vi "DefensorManMark.vi"(8 "AI Parameters":T1={"GotoKick"={"Dist do cone a frente"=150.0, "attacker farback"=1500.0, "Perto"=300.0, "min dist to kick"=150.0, "kick eps"=0.0, "Time to transition"=0.05}, "Attacker"={"CC chute"=0.09, "CC passe"=0.045, "Kick Force"=100.0, "D ball-robot Kick"=200.0, "D ball-robot Pass"=0.3}, "Defender"={"D max"=1700.0, "Vel p/ robô av"=1000.0, "Kick Force"=100.0, "D atk-def"=0.0, "D farback"=0.0}, "Timeout"={"Field/v in x"=6.0, "Dist Robots"=300, "Dist up in y"=300}, "Pose Striker"={"dist"=200.0, "Numeric"=-4.0, "dist 2"=200.0}, "Dist Stop"=300.0, "Distance when ball out"=200, "D central gap "=150.0, "T pass"=0.0, "Force ++"=0.0, "range kick"=0.0, "Chute alto"=TRUE, "Marcador novo"=TRUE} {"D central gap" format="%#_13g"; "Dist Stop" format="%#_13g"; "Pose Striker"."Numeric" format="%#_13g"; "Defender"."Kick Force" format="%#_13g"; "Defender"."Vel p/ robô av" format="%#_13g"; "Attacker"."D ball-robot Kick" format="%#_13g"; "Attacker"."Kick Force" format="%#_13g"; "Attacker"."CC passe" format="%#_13g"; "Attacker"."CC chute" format="%#_13g"; "GotoKick"."kick eps" format="%#_13g"; "GotoKick"."min dist to kick" format="%#_13g"; "GotoKick"."Perto" format="%#_13g"; "GotoKick"."attacker farback" format="%#_13g"; "GotoKick"."Dist do cone a frente" format="%#_13g"}, 9 "Robot in":T3={"id"=5, "function"=enum."Attacker", "x"=-1842.5054931640625, "y"=520.60986328125, "orientation"=-2.7555055618286133, "v_tangent"=0.0, "v_normal"=0.0, "v_ang"=0.0, "kick_x"=0.0, "kick_z"=0.0, "dribble"=FALSE, "Timestamp"=timestamp(2082758857.4639893 s since 1904-01-01), "estimatives"={"est_v_tangent"=0.0, "est_v_normal"=0.0, "est_vx"=0.0, "est_vy"=0.0, "Pos Robot Est"=[]}, "dest_x_kick"=0.0, "dest_y_kick"=0.0, "Gap Coord"=[], "States"=enum."GoToTangent", "Path "=[], "Path  Smooth"=[], "Dest"=[]}, 10 "Field Size in":T9, 11 "IA Input":T2={"our_robots"=[], "enemy_robots"=[], "balls"=[], "geometry"={"line_width"=0, "field_length"=0, "field_width"=0, "boundary_width"=0, "referee_width"=0, "goal_width"=0, "goal_depth"=0, "goal_wall_width"=0, "center_circle_radius"=0, "defense_radius"=0, "defense_stretch"=0, "free_kick_from_defense_dist"=0, "penalty_spot_from_field_line_dist"=0, "penalty_line_from_spot_dist"=0}, "IA Judge"={"stage"="", "command"="", "our_goalie_id"=0.0, "enemy_goalie_id"=0.0, "command enum"=enum."Halt", "Time"=enum."Azul"}, "Received Timestamp"=timestamp(0 s since 1904-01-01), "Events"={"Touch"=FALSE, "Ball out"=FALSE, "id touch"=0.0, "Ball out of \nVision"=FALSE, "Ball inside \nGoalie area"=FALSE, "Robot not responding"=FALSE, "Robots responding status"=[1.0, 1.0, 1.0, 1.0, 1.0, 1.0], "Enemy Ball \nPossession"=FALSE, "Pass State"=FALSE, "id end of pass"=0.0, "Kick"=FALSE, "Id ini Possession"=0.0, "Ball Possesion"=FALSE, "Id Possesion"=0.0}}) -> (2 "Robot out":T3={"id"=0, "function"=enum."Attacker", "x"=0.0, "y"=0.0, "orientation"=0.0, "v_tangent"=0.0, "v_normal"=0.0, "v_ang"=0.0, "kick_x"=0.0, "kick_z"=0.0, "dribble"=FALSE, "Timestamp"=timestamp(0 s since 1904-01-01), "estimatives"={"est_v_tangent"=0.0, "est_v_normal"=0.0, "est_vx"=0.0, "est_vy"=0.0, "Pos Robot Est"=[]}, "dest_x_kick"=0.0, "dest_y_kick"=0.0, "Gap Coord"=[], "States"=enum."GoToTangent", "Path "=[], "Path  Smooth"=[], "Dest"=[]}, 3 "id do inimigo\nmais perigoso":u32)   [LabVIEW 2017]
uses:
  Core/Field Size.ctl
  Core/AI Robot.ctl
  Functions Enum.ctl
  AttackerStates.ctl
  Path Planning/RRT/PathDests.ctl
  Path Planning/RRT/PathDest.ctl
  Core/AI Input.ctl
  Core/AI Ball.ctl
  Core/AI Judge.ctl
  Command Enum.ctl
  Util/Events/Events.ctl
  AI Parameters.ctl
  <vilib>/Analysis/_algsub.llb/Real Vector Norm.vi
  <vilib>/Analysis/NI_AALPro.lvlib
panel:
  in  "farback striker":dbl=500.0 format="%#_13g"
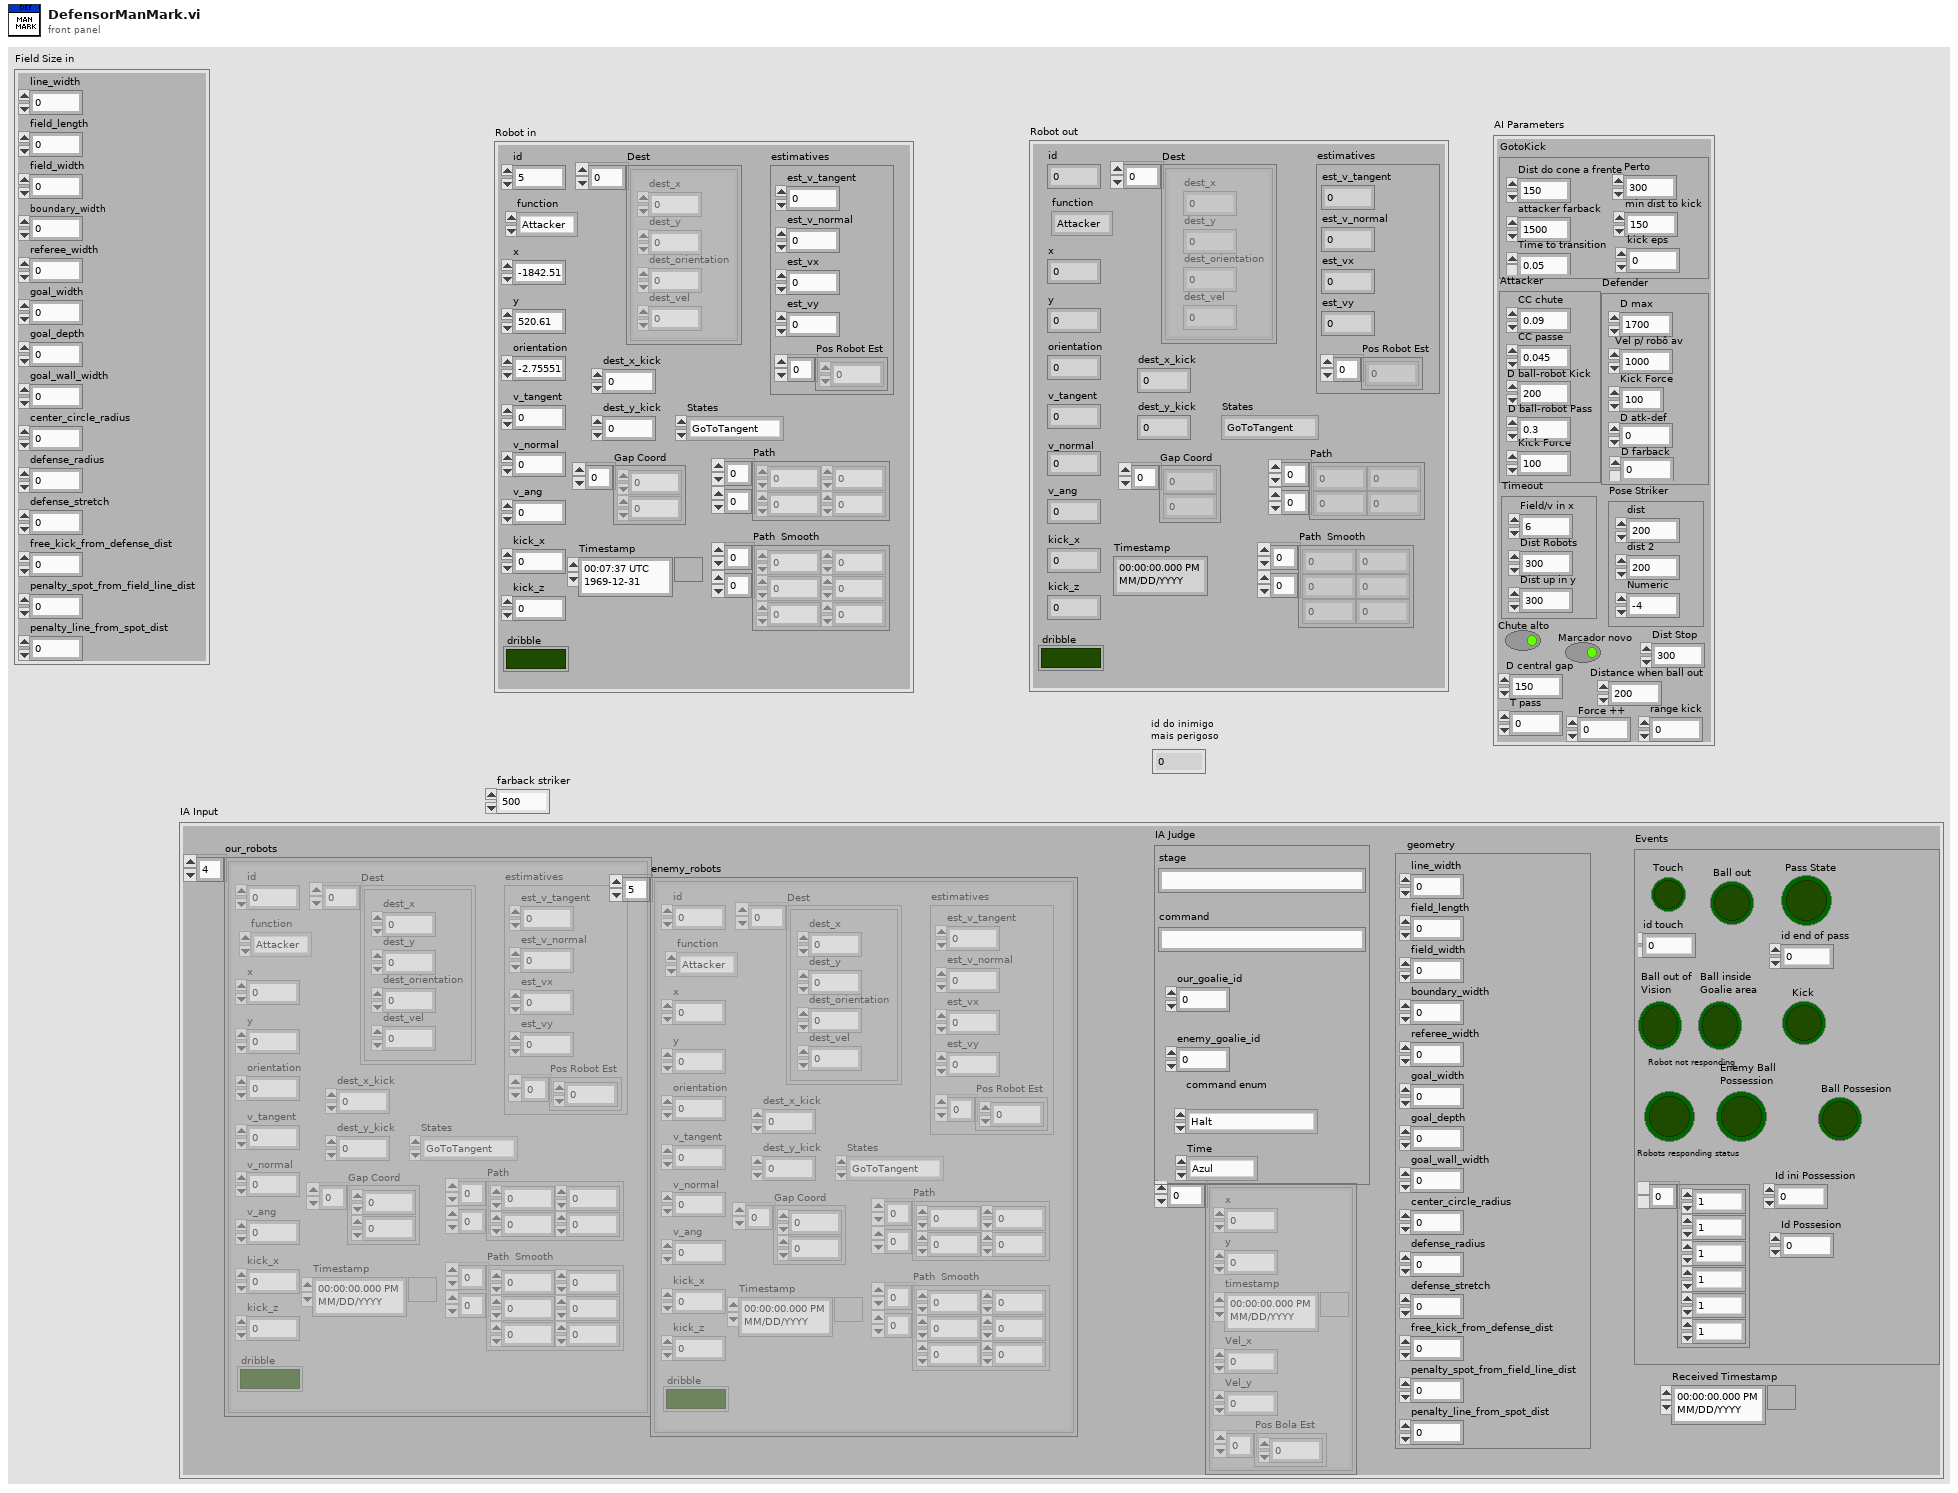
[diagram p1: front panel]
types:
  T1 = typedef "AI Parameters.ctl" = cluster{"GotoKick":cluster{"Dist do cone a frente":dbl, "attacker farback":dbl, "Perto":dbl, "min dist to kick":dbl, "kick eps":dbl, "Time to transition":dbl}, "Attacker":cluster{"CC chute":dbl, "CC passe":dbl, "Kick Force":dbl, "D ball-robot Kick":dbl, "D ball-robot Pass":dbl}, "Defender":cluster{"D max":dbl, "Vel p/ robô av":dbl, "Kick Force":dbl, "D atk-def":dbl, "D farback":dbl}, "Timeout":cluster{"Field/v in x":dbl, "Dist Robots":u32, "Dist up in y":u32}, "Pose Striker":cluster{"dist":dbl, "Numeric":dbl, "dist 2":dbl}, "Dist Stop":dbl, "Distance when ball out":i32, "D central gap ":dbl, "T pass":dbl, "Force ++":dbl, "range kick":dbl, "Chute alto":bool, "Marcador novo":bool}
  T2 = typedef "AI Input.ctl" = cluster{"our_robots":T3[], "enemy_robots":T3[], "balls":T8[], "geometry":T9, "IA Judge":T10, "Received Timestamp":timestamp, "Events":T12}
  T3 = typedef "AI Robot.ctl" = cluster{"id":u32, "function":T4, "x":dbl, "y":dbl, "orientation":dbl, "v_tangent":dbl, "v_normal":dbl, "v_ang":dbl, "kick_x":dbl, "kick_z":dbl, "dribble":bool, "Timestamp":timestamp, "estimatives":cluster{"est_v_tangent":dbl, "est_v_normal":dbl, "est_vx":dbl, "est_vy":dbl, "Pos Robot Est":dbl[]}, "dest_x_kick":dbl, "dest_y_kick":dbl, "Gap Coord":dbl[], "States":T5, "Path ":dbl[][], "Path  Smooth":dbl[][], "Dest":T6}
  T4 = typedef "Functions Enum.ctl" = enum16{"Attacker", "Goalie", "Defender", "Striker", "Goto 0", "Dummy", "Kicker", "ZigZag"}
  T5 = typedef "AttackerStates.ctl" = enum16{"Pass", "GoToTangent", "BallGetting", "GoToKick", ""}
  T6 = typedef "PathDests.ctl" = T7[]
  T7 = typedef "PathDest.ctl" = cluster{"dest_x":dbl, "dest_y":dbl, "dest_orientation":dbl, "dest_vel":dbl}
  T8 = typedef "AI Ball.ctl" = cluster{"x":dbl, "y":dbl, "timestamp":timestamp, "Vel_x":dbl, "Vel_y":dbl, "Pos Bola Est":dbl[]}
  T9 = typedef "Field Size.ctl" = cluster{"line_width":u32, "field_length":u32, "field_width":u32, "boundary_width":u32, "referee_width":u32, "goal_width":u32, "goal_depth":u32, "goal_wall_width":u32, "center_circle_radius":u32, "defense_radius":u32, "defense_stretch":u32, "free_kick_from_defense_dist":u32, "penalty_spot_from_field_line_dist":u32, "penalty_line_from_spot_dist":u32}
  T10 = typedef "AI Judge.ctl" = cluster{"stage":string, "command":string, "our_goalie_id":dbl, "enemy_goalie_id":dbl, "command enum":T11, "Time":enum16{"Azul", "Amarelo"}}
  T11 = typedef "Command Enum.ctl" = enum16{"Halt", "Stop", "Force Start", "PKA Normal Start", "Prepare Kickoff Ally", "PKE Normal Start", "Prepare Kickoff Enemy", "Prepare Penalty Ally", "PPA Normal Start", "Prepare Penalty Enemy", "PPE Normal Start", "Direct Free Enemy", "Direct Free Ally", "Indirect Free Enemy", "Indirect Free Ally", "Timeout Enemy", "Timeout Ally", "Goal Enemy", "Goal Ally", "Ball Placement Enemy", "Ball Placement Ally", "Normal Half Time", "Extra Time Break", "Extra Half Time", "None", "Post Game"}
  T12 = typedef "Events.ctl" = cluster{"Touch":bool, "Ball out":bool, "id touch":dbl, "Ball out of \nVision":bool, "Ball inside \nGoalie area":bool, "Robot not responding":bool, "Robots responding status":dbl[], "Enemy Ball \nPossession":bool, "Pass State":bool, "id end of pass":dbl, "Kick":bool, "Id ini Possession":dbl, "Ball Possesion":bool, "Id Possesion":dbl}
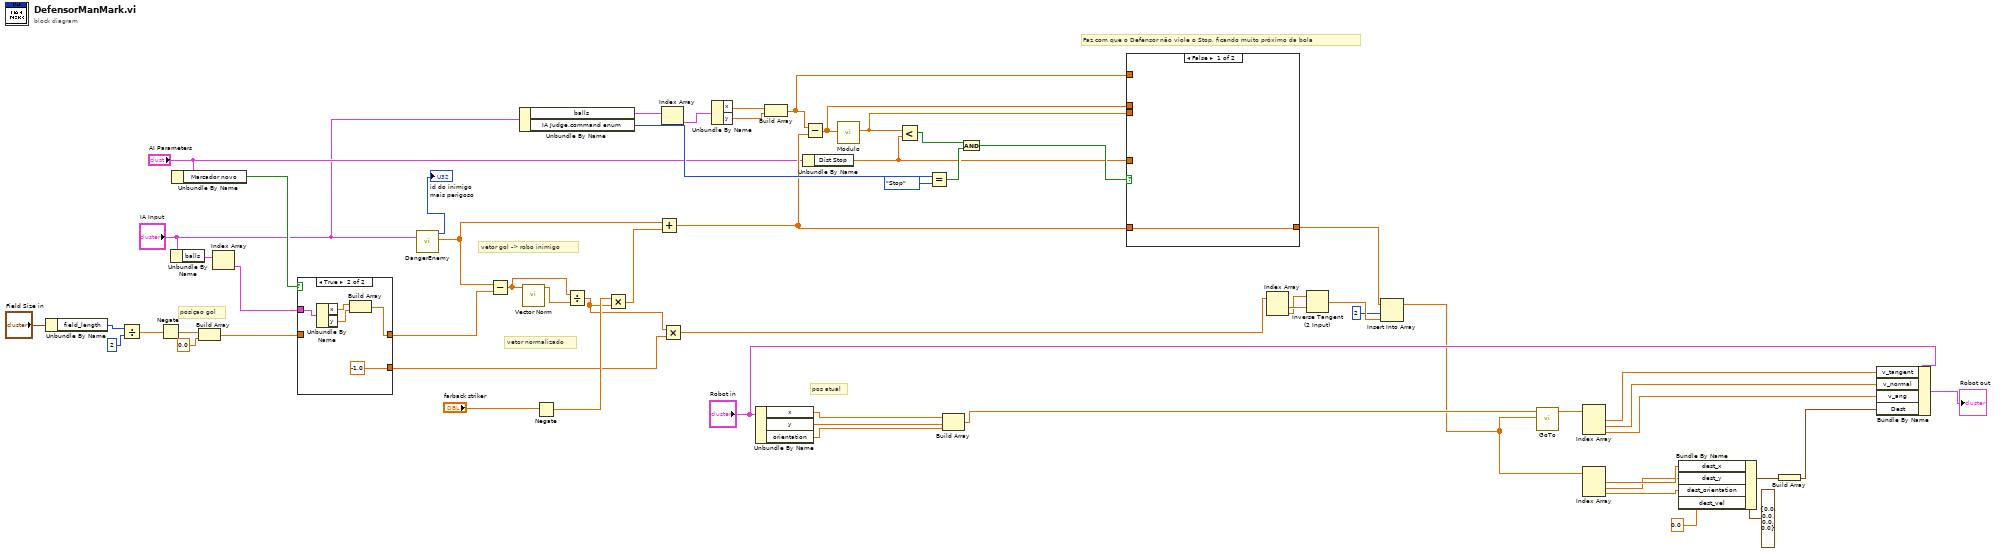
[diagram p0: block diagram]
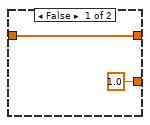
[diagram p2: hidden frame]
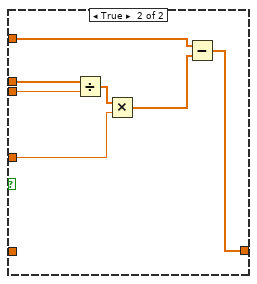
[diagram p3: hidden frame]
diagram:
  # "Faz com que o Defensor não viole o Stop, ficando muito próximo da bola"
  # "pos atual"
  # "vetor normalizado"
  # "vetor gol -> robo inimigo"
  # "posiçao gol"
  n1 = Unbundle By Name("Field Size in") -> ("field_length"=w59:u32)
  n2 = Divide(x=w59, y=u32 2) -> (x/y=w57:dbl)
  n3 = Negate(x=w57) -> (-x=w56:dbl)
  n4 = Unbundle By Name("IA Input") -> ("balls"=w16:T8[])
  n5 = Unbundle By Name("AI Parameters") -> ("Marcador novo"=w18:bool)
  n6 = Build Array(w56, 0.0 ("element")) -> (w21:dbl[])
  n7 = Index Array(array=w16) -> (element=w15:T8)  [unwired: 1 in]
  n8 = case shown="True" w18 {
    tunnel: [w62 w64] -> w20
    tunnel: w21 -> [w62 _]
    tunnel: w15 -> [_ w67]
    tunnel: [1.0 -1.0] -> w10
    frame False {
    }
    frame True {
      n9 = Unbundle By Name(w67) -> ("x"=w66:dbl, "y"=w65:dbl)
      n10 = Build Array(w66, w65) -> (w64:dbl[])
    }
  }
  n11 = call "DangerEnemy.vi"("IA Input"="IA Input") -> ("Pos do inimigo\nperigoso"=w1:dbl[], "id do inimigo\nmais perigoso"=→"id do inimigo\nmais perigoso":u32)  [unwired: 7 in, 2 out]
  n12 = Subtract(x=w1, y=w20) -> (x-y=w53:dbl[])
  n13 = Unbundle By Name("IA Input") -> ("balls"=w35:T8[], "IA Judge.command enum"=w29:T11)
  n14 = call-poly <vilib>:"Vector Norm.vi"("Input Vector"=w53) -> ("norm"=w54:dbl)  [unwired: 9 in, 1 out]
  n15 = Negate(x="farback striker") -> (-x=w37:dbl)
  n16 = Divide(x=w53, y=w54) -> (x/y=w12:dbl[])
  n17 = Multiply(x=w37, y=w12) -> (x*y=w36:dbl[])
  n18 = Add(x=w1, y=w36) -> (x+y=w26:dbl[])
  n19 = Index Array(array=w35) -> (element=w34:T8)  [unwired: 1 in]
  n20 = Multiply(x=w12, y=w10) -> (x*y=w11:dbl[])
  n21 = Unbundle By Name(w34) -> ("x"=w33:dbl, "y"=w32:dbl)
  n22 = Unbundle By Name("Robot in") -> ("x"=w48:dbl, "y"=w47:dbl, "orientation"=w46:dbl)
  n23 = Build Array(w33, w32) -> (w23:dbl[])
  n24 = Unbundle By Name("AI Parameters") -> ("Dist Stop"=w24:dbl)
  n25 = Subtract(x=w23, y=w26) -> (x-y=w22:dbl[])
  n26 = call "Modulo.vi"("2D vector"=w22) -> ("Modulo"=w25:dbl)  [unwired: 10 in]
  n27 = Less?(x=w25, y=w24) -> (x < y?=w31:bool)
  n28 = Equal?(x=w29, y=Command_Enum."Stop") -> (x = y?=w30:bool)
  n29 = Build Array(w48, w47, w46) -> (w45:dbl[])
  n30 = And(x=w31, y=w30) -> (x .and. y?=w27:bool)
  n31 = case shown="False" w27 {
    tunnel: [w68 w70] -> w14
    tunnel: w26 -> [w68 _]
    tunnel: w25 -> [_ w75]
    tunnel: w24 -> [_ w73]
    tunnel: w23 -> [_ w72]
    tunnel: w22 -> [_ w69]
    frame False {
    }
    frame True {
      n32 = Divide(x=w69, y=w75) -> (x/y=w74:dbl[])
      n33 = Multiply(x=w74, y=w73) -> (x*y=w71:dbl[])
      n34 = Subtract(x=w72, y=w71) -> (x-y=w70:dbl[])
    }
  }
  n35 = Index Array(array=w11) -> (element #1=w52:dbl, element #2=w51:dbl)  [unwired: 2 in]
  n36 = Inverse Tangent (2 Input)(1:w52, 2:w51) -> (0:w50:dbl)
  n37 = Insert Into Array(array=w14, index=2, new element=w50) -> (w13:dbl[])
  n38 = call "GoTo.vi"("Target"=w13, "Position"=w45) -> ("Output\nVelocity"=w44:dbl[])  [unwired: 8 in, 1 out]
  n39 = Index Array(array=w44) -> (element #1=w43:dbl, element #2=w42:dbl, element #3=w41:dbl)  [unwired: 3 in]
  n40 = Index Array(array=w13) -> (element #1=w5:dbl, element #2=w4:dbl, element #3=w3:dbl)  [unwired: 3 in]
  n41 = Bundle By Name(cluster=T7 {"dest_x"=0.0, "dest_y"=0.0, "dest_orientation"=0.0, "dest_vel"=0.0} ("Dest"), "dest_x"=w5, "dest_y"=w4, "dest_orientation"=w3, "dest_vel"=0.0) -> (w8:T7)
  n42 = Build Array(w8) -> (w6:T7[])
  n43 = Bundle By Name(cluster="Robot in", "v_tangent"=w43, "v_normal"=w42, "v_ang"=w41, "Dest"=w6) -> (→"Robot out":T3)
